vi "Edge Detection.vi"() -> ()   [LabVIEW 2016]
doc: "This example shows how to use the Edge Tool in NI Vision. The Edge Tool finds edges (or sharp transitions in the pixels values) along a given line or ROI profile. The Edge Tool is a precursor function to many of the gauging and inspection tasks. For example, the location of the edges found along a line profile across an object can interpreted as the boundaries of the object whose dimensions have to be measured for a gauging application or the presence of a crack in the surface of an object for an inspection application."
uses:
  <vilib>/userdefined/High Color/IMAQdx.ctl
  <vilib>/vision/NI_Vision_Development_Module.lvlib
  <vilib>/vision/driver/NI_Vision_Acquisition_Software.lvlib
panel:
  out "Line Equation":cluster{"A":dbl, "B":dbl, "C":dbl} {"C" format="%.2f"; "B" format="%.2f"; "A" format="%.2f"}
  out "Number of Edges Detected":i32
  in  "Process":u16(ring) items=["Get First Edge", "Get First + Last Edge", "Get All Edges", "Get Best Edge"]
  in  "Edge Options":T1={"Edge Polarity"=2, "Kernel Size"=37, "Width"=5, "Minimum Edge Strength"=10.0, "Interpolation Type"=0, "Data Processing Method"=1} {"Data Processing Method" items=["Average", "Median"]; "Interpolation Type" items=["Zero Order"=0, "Bilinear"=1, "Bilinear Fixed"=4]; "Minimum Edge Strength" min=0.0 max=255.0 format="%.2g"; "Width" min=1 step=2; "Kernel Size" min=3 step=2; "Edge Polarity" items=["All Edges", "Rising Edges", "Falling Edges"]}
  out "Gradient Information":dbl[](graph)
  out "Image":T2(plugin-control)
  out "Line Profile":cluster{"x0":sgl, "dx":sgl, "Pixels Line":sgl[]}(graph)
  in  "Stop":bool
  # "Overview: Demonstrates how to use the IMAQ Edge Tool function to find edges along a Region of Interest (ROI).\nRequirements: Vision Development Software.\nInstructions:\n1. Run the VI.\n2. Draw a ROI in the image or change the Process or Edge Options to see the edges detected along the ROI."
  # "Ax + By + C = 0"
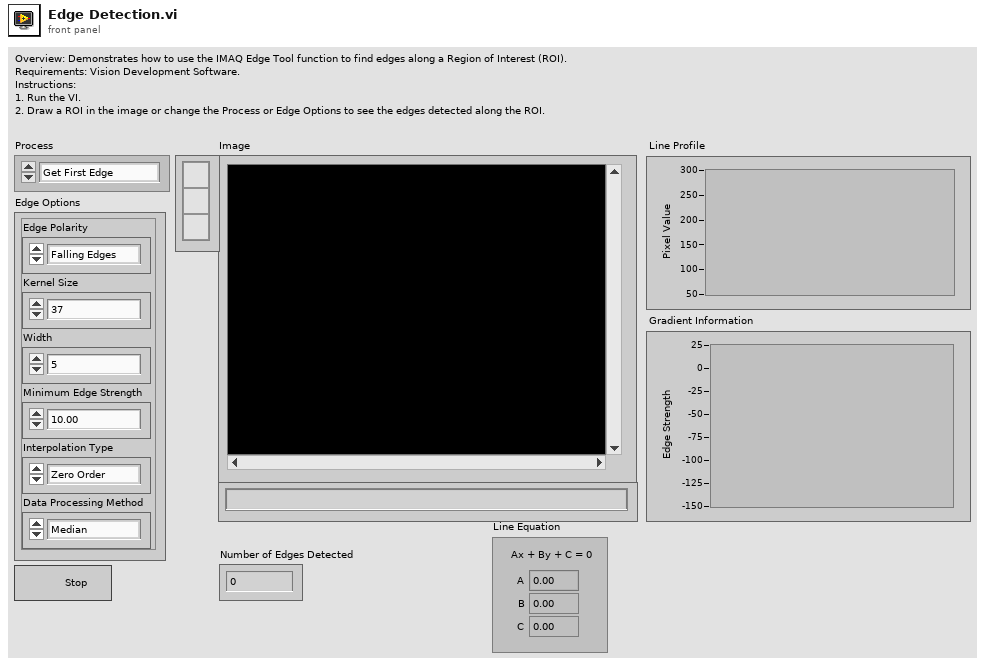
[diagram p1: front panel]
types:
  T1 = cluster{"Edge Polarity":u16, "Kernel Size":u32, "Width":u32, "Minimum Edge Strength":dbl, "Interpolation Type":u16, "Data Processing Method":u16}
  T2 = typedef "IMAQ Image.ctl" = refnum<image>
  T3 = typedef "IMAQ Line" = cluster{"Start X":i32, "Start Y":i32, "End X":i32, "End Y":i32}
  T4 = typedef "Image Type" = u32
  T5 = typedef "IMAQdx.ctl" = refnum<k21>
  T6 = typedef "ROI Descriptor" = cluster{"Global Rectangle":i32[], "Contours":cluster{"ID":enum32{"External", "Internal"}, "Type":u32, "Coordinates":i32[]}[]}
  T7 = cluster{"Global Rectangle":i32[], "Contours":cluster{"Contour Type":u32, "ROI Type":u32, "Points":i32[]}[]}
  T8 = typedef "Edge New.ctl" = cluster{"Location (Pixel)":cluster{"X":sgl, "Y":sgl}, "Location (Real-World)":cluster{"X":sgl, "Y":sgl}, "Distance (Pixel)":dbl, "Distance (Real-World)":dbl, "Strength":dbl, "Noise":dbl, "Rising?":bool}
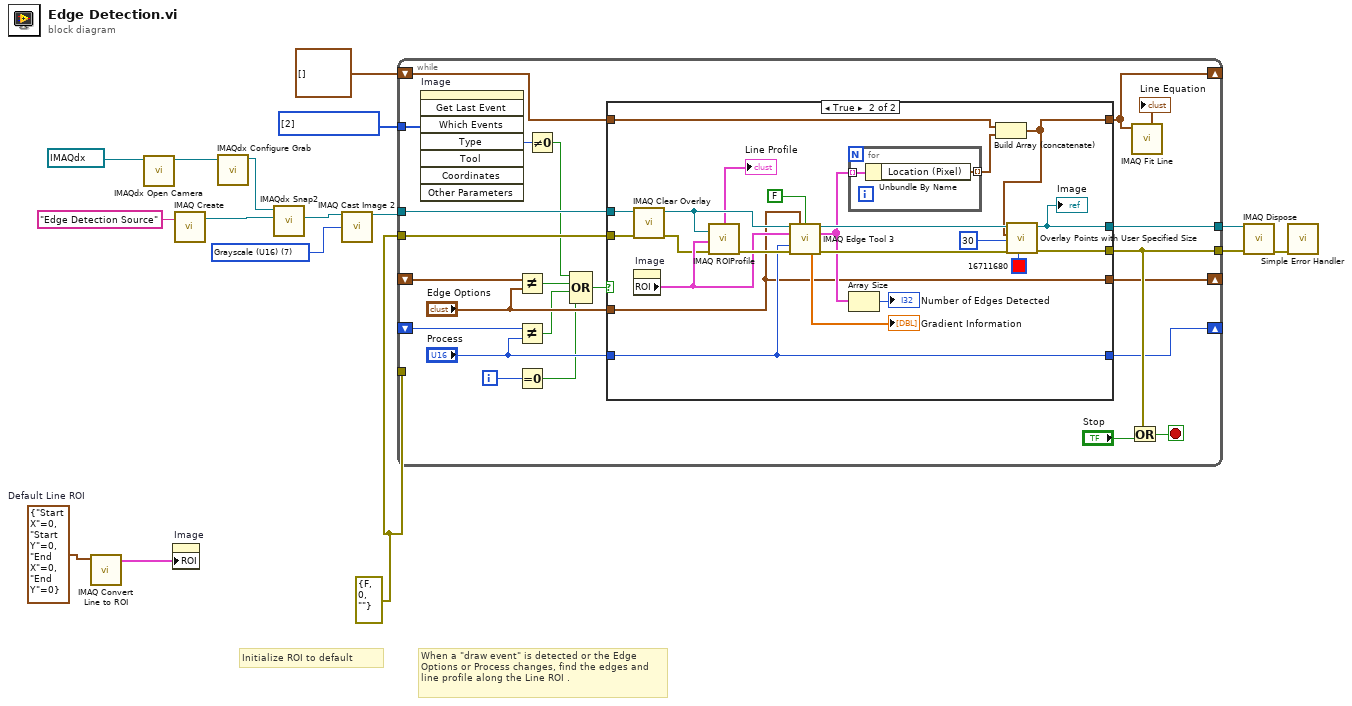
[diagram p0: block diagram]
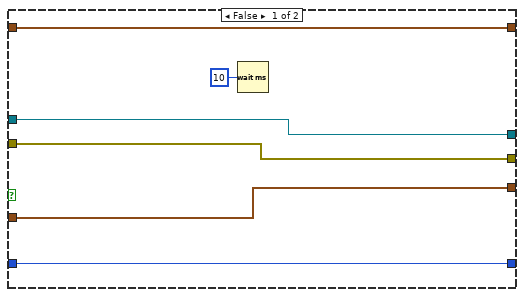
[diagram p2: hidden frame]
diagram:
  w1 = T3 {"Start X"=0, "Start Y"=0, "End X"=0, "End Y"=0}  # Default Line ROI
  w3 = errorcluster {"status"=FALSE, "code"=0, "source"=""} ("error out")
  w4 = T4 7 items=["Grayscale (U8)", "Grayscale (I16)", "Grayscale (SGL)", "Complex (CSG)", "RGB (U32)", "HSL (U32)", "RGB (U64)", "Grayscale (U16)"] ("Image Type")
  w12 = i32[] [2] items=["No  event", "Click event", "Draw event", "Move event", "Size event", "Scroll event", "Activate event", "Close event", "Double click event"] ("Events list (all)")
  # "Initialize ROI to default"
  # "When a \"draw event\" is detected or the Edge Options or Process changes, find the edges and line profile along the Line ROI ."
  n1 = call "IMAQ Convert Line to ROI"("Line"=w1) -> ("ROI Descriptor"=w2:T6)  [unwired: 8 in, 1 out]
  n2 = call <vilib>:"IMAQdx Open Camera.vi"("Session In"=T5 "cam0") -> ("Session Out"=w9:T5)  [unwired: 9 in, 1 out]
  n3 = property on="Image" class="ImageControl"("ROI"=w2) -> ()  [unwired: 2 in, 2 out]
  n4 = call "IMAQ Create"("Image Name"="Edge Detection Source") -> ("New Image"=w8:T2)  [unwired: 4 in, 1 out]
  n5 = call <vilib>:"IMAQdx Configure Grab.vi"("Session In"=w9) -> ("Session Out"=w7:T5)  [unwired: 9 in, 1 out]
  n6 = call <vilib>:"IMAQdx Snap2.vi"("Image In"=w8, "Session In"=w7) -> ("Image Out"=w6:T2)  [unwired: 7 in, 2 out]
  n7 = call "IMAQ Cast Image 2"("Image Src"=w6, "Image Type"=w4) -> ("Image Dst Out"=w5:T2)  [unwired: 12 in, 1 out]
  n8 = while {
    tunnel: w5 -> [w38]
    tunnel: w3 -> [w39]
    tunnel: [w34] -> w15
    tunnel: [w35] -> w14
    tunnel: w12 -> [w33]
    shift-right: [w20] -> _
    shift-left: _ -> [w30]
    shift-right: [w21] -> _
    shift-left: _ -> [w28]
    tunnel: w3 -> [_]
    shift-right: [w18] -> _
    shift-left: cluster{"X":sgl, "Y":sgl}[] [] -> [w19]
    i -> [w31]
    stop <- w36 stop-if-true
    n9 = invoke on="Image" class="ImageControl" method="Get Last Event"("Which Events"=w33) -> ("Type"=w32:i32)  [unwired: 7 in, 7 out]
    n10 = Not Equal?(x=w30, y="Edge Options") -> (x != y?=w26:bool)
    n11 = Not Equal?(x=w28, y="Process") -> (x != y?=w25:bool)
    n12 = Equal To 0?(x=w31) -> (x = 0?=w24:bool)
    n13 = Not Equal To 0?(x=w32) -> (x != 0?=w23:bool)
    n14 = Compound Arithmetic op=OR(w23, w26, w25, w24) -> (w22:bool)
    n15 = case shown="True" w22 {
      tunnel: w39 -> [w44 w57]
      tunnel: w38 -> [w45 w56]
      tunnel: [w45 w59] -> w35
      tunnel: [w44 w63] -> w34
      tunnel: "Edge Options" -> [w42 w50]
      tunnel: "Process" -> [w41 w52]
      tunnel: [w41 w52] -> w21
      tunnel: [w42 w50] -> w20
      tunnel: w19 -> [w40 w49]
      tunnel: [w40 w47] -> w18
      frame False {
        n16 = Wait (ms)(milliseconds to wait=u32 10) -> ()  [unwired: 1 out]
      }
      frame True {
        n17 = call "IMAQ Clear Overlay"("error in (no error)"=w57, "Image"=w56) -> ("error out"=w54:errorcluster, "Image Out"=w55:T2)  [unwired: 8 in]
        n18 = property on="Image" class="ImageControl"() -> ("ROI"=w58:T7)  [unwired: 2 in, 2 out]
        n19 = call "IMAQ ROIProfile"("error in (no error)"=w54, "ROI Descriptor"=w58, "Image"=w55) -> ("error out"=w65:errorcluster, "ROI Graph"=→"Line Profile":cluster{"x0":sgl, "dx":sgl, "Pixels Line":sgl[]})  [unwired: 1 in, 3 out]
        n20 = call "IMAQ Edge Tool 3"("Image"=w55, "Edge Options"=w50, "Optimized Mode"=FALSE, "ROI Descriptor"=w58, "Process"=w52, "error in (no error)"=w65) -> ("Image (duplicate)"=w62:T2, "Edge Information"=w61:T8[], "Gradient Values"=→"Gradient Information":dbl[], "error out"=w64:errorcluster)  [unwired: 5 in, 1 out]
        n21 = for {
          tunnel: w61 -> [w69] mode=indexing
          tunnel: [w68] -> w48 mode=indexing
          n22 = Unbundle By Name(w69) -> ("Location (Pixel)"=w68:cluster{"X":sgl, "Y":sgl})
        }
        n23 = Array Size(array=w61) -> (size(s)=→"Number of Edges Detected":i32)
        n24 = Build Array (concatenate)(w49, w48) -> (w47:cluster{"X":sgl, "Y":sgl}[])
        n25 = call "Overlay Points with User Specified Size.vi"("Color"=u32 16711680, "error in"=w64, "Point Diameter (5)"=30, "Points"=w47, "Image In"=w62) -> ("error out"=w63:errorcluster, "Image Out"=w59:T2)  [unwired: 5 in]
        "Image" <- w59
      }
    }
    n26 = Or(x=w34, y="Stop") -> (x .or. y?=w36:bool)
    n27 = call "IMAQ Fit Line"("Points"=w18) -> ("Line Equation"=→"Line Equation":cluster{"A":dbl, "B":dbl, "C":dbl})  [unwired: 5 in, 5 out]
  }
  n28 = call "IMAQ Dispose"("Image"=w14, "error in (no error)"=w15) -> ("error out"=w13:errorcluster)  [unwired: 4 in]
  n29 = call <vilib>:"Simple Error Handler.vi"("error in (no error)"=w13) -> ()  [unwired: 4 in, 5 out]
